vi "AmpCal.vi"(4 "Burst Ct":i8[](array[numeric])=[1, 3, 5, 10, 20], 6 "CA Threshold":i16=62, 8 "File Name In":string, 9 "Voltage Steps":sgl[](array[numeric])=[100.0] format="%_3g", 10 "Motion Settings":T1={"No Motion?"=FALSE, "Motion System"=enum."NI 735x", "Motion Bd ID"=1, "Motion Profile"="SMAC1", "# Axis"=1, "Reverse Z axis?"=TRUE, "SMAC Axis"=0, "scan pair"=enum."y-(x) scan", "RT fps"=6.0, "Steps per mm"=[1000, 1000, 1000, 1000], "Motor Parameters"={"velocity ct/s"=[10000.0, 10000.0, 10000.0, 50000.0], "accel ct/s^2"=[50000.0, 50000.0, 50000.0, 200000.0]}, "One Way Scan"=FALSE, "Reverse One Way Scan"=FALSE, "Global Position (mm)"=[], "Plane"=0, "Distance between\nscan lines (um)"=0.0, "Distance between\nscan planes (um)"=0.0, "number of scan planes"=1, "Total steps in line"=0, "Xtra plane\ndistance  (um)"=100, "Xtra planes "=1, "Add Axis"=FALSE, "overshoot cts"=200, "BKPT Shift"=0, "Scan Start Time (ms)"=0, "ESP VISA"="GPIB::1::INSTR", "3rd Axis"=1, "GL Ref Out"=refnum, "Galil Address"=""} {"3rd Axis" items=["x", "y", "z", "w"]; "Xtra planes" min=1; "Xtra plane\ndistance  (um)" min=0; "Distance between\nscan planes (um)" format="%.2f"; "Distance between\nscan lines (um)" format="%.2f"; "SMAC Axis" items=["None"=0, "Axis 1"=1, "Axis 2"=2, "Axis 3"=3, "Axis 4"=4, "Axis 5"=5, "Axis 6"=6, "Axis 7"=7, "Axis 8"=8, "Vector Space 1"=17, "Vector Space 2"=18, "Vector Space 3"=19, "Vector Space 4"=20]; "Motion Bd ID" min=1 max=32 step=1}, 11 "Digitizer Settings":T5={"Digitizer delay (us) "=0.0, "rf points per line"=2048, "lines per plane"=128, "Samp Rate (Hz)"=100000000.0, "Additional dig delay (us)"=0.0, "Voltage Scale"=0.4, "Pre-Looks"=0, "Offset delay (us)"=0.0, "bits A/D"=8, "Avg Num"=1, "DigTimeOut"=5.0, "Rel Dig Delay"=0.0, "Dig Ch"=0, "LeCroyCluster"={"LeCroy Channels"=[TRUE, FALSE, FALSE, FALSE], "LC read pt offset"=0.0, "Sweep Avg"=FALSE}, "Main Digitizer"=enum."NI Digitizer", "Dig Config"=enum."Single channel", "Digitizer ID Cluster"={"Acqiris/Alazar/SP ID"=[], "NI Instr Handles"=[], "LeCroy VISA"="", "GaGe Handle"={"Handle"=0, "Sample size"=0, "Resolution"=0, "Offset"=0, "Channels"=0, "Boards"=0}, "ATS Ref"="ATS9350", "Acqiris Address"=["PCI::INSTR0"], "ADQRef"=refnum, "adq_cu_ptr"=refnum}, "Trigger Settings"={"Trig Source"=1, "Trig Coupling"=0, "Trig Slope"=0, "Level (mV)"=1500.0}, "Bulk Acq"=FALSE, "Bulk Start Indexes"=[], "Data Ref RF"=refnum, "NI ID/Channel"=[], "Total Dig CH"=5, "Xtra Ann Trig delay (us)"=10.0, "Fix Z Delay?"=FALSE, "One Way Transmission?"=FALSE, "Data Ref Log"=refnum} {"Trigger Settings"."Trig Slope" items=["Positive", "Negative"]; "Trigger Settings"."Level (mV)" format="%.2f"; "Trigger Settings"."Trig Coupling" items=["DC 1 MOhm", "AC 1 MOhm", "DC 50 Ohm", "AC 50 Ohm"]; "Trigger Settings"."Trig Source" items=["Chan 1", "External"]; "Rel Dig Delay" format="%.2f"; "DigTimeOut" format="%.2f"; "Avg Num" min=1; "Offset delay (us)" format="%.2f"; "Additional dig delay (us)" format="%.2f"; "Digitizer delay (us)" format="%.2f"}) -> (1 "Scan Params":T9, 2 "low %":dbl, 3 "clip%":dbl)   [LabVIEW 2022 SP3]
uses:
  ScanningControl/Motion Controllers/-MotionRoutines/MotionGlobals.vi
  <instrlib>/Acqiris Dx/Acqiris Dx.lvlib
  Instance           7 16Saved   Contrast .vi
  Instance           8 16Saved   Contrast .vi
  ScanningControl/Digitizers/Acqiris/-AcqirisRoutines/VScaleInfoAcq.vi
  <instrlib>/niScope/Acquire/Fetch/niScope Multi Fetch Binary 8.vi
  ScanningControl/Digitizers/NI Digitizer/-NI Digitizer VI Library/VScaleInfoNI.vi
  <vilib>/Utility/file.llb/Write To Spreadsheet File (string).vi
  <vilib>/Utility/file.llb/Read From Spreadsheet File (string).vi
  <vilib>/Utility/file.llb/Write To Spreadsheet File (I64).vi
  ScanningControl/Digitizers/-DigitizerRoutines/DigitizerSettings.ctl
  ScanningControl/Digitizers/-DigitizerRoutines/DigitizerID.ctl
  ScanningControl/Digitizers/-DigitizerRoutines/Digitizer.ctl
  ScanningControl/Motion Controllers/NI_controller/-NI_MotionRoutines/MotionSys.ctl
  ScanningControl/Motion Controllers/-MotionRoutines/ScanAxis.ctl
  ScanningControl/Motion Controllers/NI_controller/-NI_MotionRoutines/MotionParameters.ctl
  ScanningControl/Digitizers/-DigitizerRoutines/DigConfig.ctl
  ScanningControl/Motion Controllers/-MotionRoutines/3rdAxis.ctl
  C:/Windows/System32/ADQAPI_dotNet_helper.dll
panel:
  out "try":i32=100
  # "1-D and 2-D B scan settings"
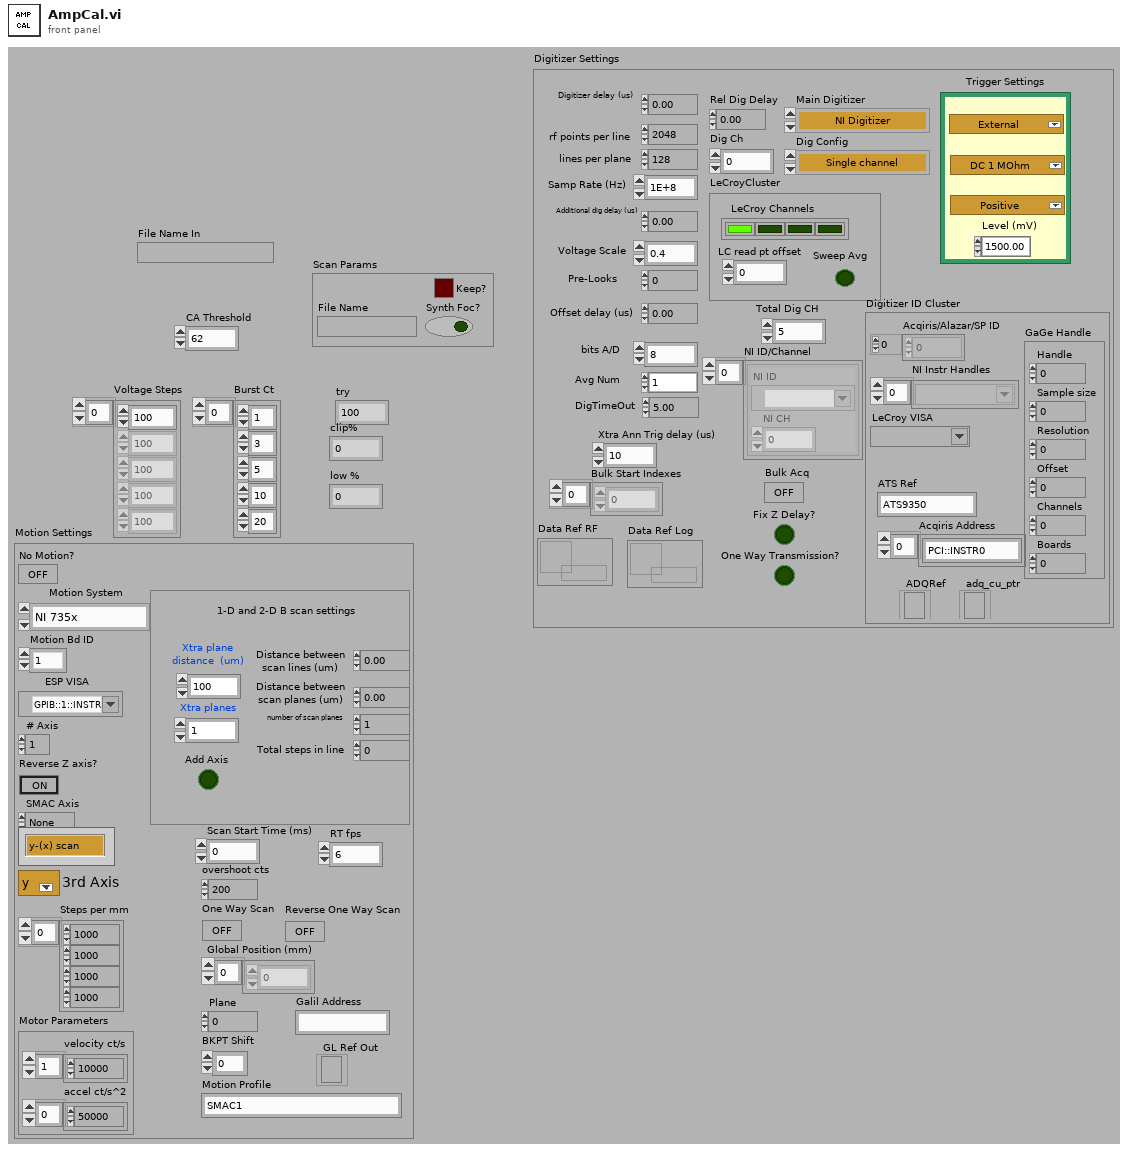
[diagram p1: front panel]
types:
  T1 = typedef "MotionParameters.ctl" = cluster{"No Motion?":bool, "Motion System":T2, "Motion Bd ID":u8, "Motion Profile":string, "# Axis":i8, "Reverse Z axis?":bool, "SMAC Axis":u16, "scan pair":T3, "RT fps":sgl, "Steps per mm":i32[], "Motor Parameters":cluster{"velocity ct/s":dbl[], "accel ct/s^2":dbl[]}, "One Way Scan":bool, "Reverse One Way Scan":bool, "Global Position (mm)":dbl[], "Plane":i32, "Distance between\nscan lines (um)":sgl, "Distance between\nscan planes (um)":sgl, "number of scan planes":i32, "Total steps in line":i32, "Xtra plane\ndistance  (um)":i32, "Xtra planes ":i32, "Add Axis":bool, "overshoot cts":i32, "BKPT Shift":i32, "Scan Start Time (ms)":u32, "ESP VISA":refnum<visa-resource-name>, "3rd Axis":T4, "GL Ref Out":refnum<k7>, "Galil Address":string}
  T2 = typedef "MotionSys.ctl" = enum16{"MM3000", "NI 735x", "Newport ESP", "No Motion Card", "Galil"}
  T3 = typedef "ScanAxis.ctl" = enum16{"y-(x) scan", "x-(y) scan", "z-(x) scan", "z-(y) scan", "y-(z) scan", "x-(z) scan", "w-(x) scan", "w-(y) scan", "w-(z) scan", "x-(w) scan", "y-(w) scan", "z-(w) scan"}
  T4 = typedef "3rdAxis.ctl" = u16
  T5 = typedef "DigitizerSettings.ctl" = cluster{"Digitizer delay (us) ":dbl, "rf points per line":i32, "lines per plane":i32, "Samp Rate (Hz)":dbl, "Additional dig delay (us)":dbl, "Voltage Scale":dbl, "Pre-Looks":i32, "Offset delay (us)":dbl, "bits A/D":i8, "Avg Num":i32, "DigTimeOut":sgl, "Rel Dig Delay":sgl, "Dig Ch":i32, "LeCroyCluster":cluster{"LeCroy Channels":bool[], "LC read pt offset":dbl, "Sweep Avg":bool}, "Main Digitizer":T6, "Dig Config":T7, "Digitizer ID Cluster":T8, "Trigger Settings":cluster{"Trig Source":u16, "Trig Coupling":u16, "Trig Slope":u16, "Level (mV)":dbl}, "Bulk Acq":bool, "Bulk Start Indexes":i32[], "Data Ref RF":refnum<data-value>, "NI ID/Channel":cluster{"NI ID":refnum<k15>, "NI CH":i32}[], "Total Dig CH":i32, "Xtra Ann Trig delay (us)":dbl, "Fix Z Delay?":bool, "One Way Transmission?":bool, "Data Ref Log":refnum<data-value>}
  T6 = typedef "Digitizer.ctl" = enum16{"Acqiris Digitizer", "NI Digitizer", "LeCroy", "GaGe", "AlazarTech", "No Digitizer", "Teledyne"}
  T7 = typedef "DigConfig.ctl" = enum16{"Single channel", "2 Chans w/ 2 Acqiris", "2 Chans w/ 1 Acqiris", "5-CH Pulser New", "5-CH pulser w/ ann array", "5-pass style ann array", "Empty"}
  T8 = typedef "DigitizerID.ctl" = cluster{"Acqiris/Alazar/SP ID":u32[], "NI Instr Handles":refnum<k15>[], "LeCroy VISA":refnum<visa-resource-name>, "GaGe Handle":cluster{"Handle":u32, "Sample size":u32, "Resolution":i32, "Offset":i32, "Channels":u32, "Boards":u32}, "ATS Ref":string, "Acqiris Address":string[], "ADQRef":refnum<k24>, "adq_cu_ptr":refnum<k24>}
  T9 = cluster{"File Name":string, "Keep?":bool, "Synth Foc?":bool}
  T10 = cluster{"Voltage Scale":i16, "Offset":dbl, "Coupling":u16}
  T11 = cluster{"actualSamples":i32, "absoluteInitialX":dbl, "relativeInitialX":dbl, "xIncrement":dbl, "offset":dbl, "gain":dbl, "reserved1":dbl, "reserved2":dbl}[]
  T12 = cluster{"actualSamples":i32, "absoluteInitialX":dbl, "relativeInitialX":dbl, "xIncrement":dbl, "offset":dbl, "gain":dbl, "reserved1":dbl, "reserved2":dbl}
  T13 = cluster{"Voltage Scale":dbl, "Offset":dbl, "Coupling":u16}
  T14 = cluster{sgl, "Gain [dB]  ":sgl, "Atten (dB)":sgl}
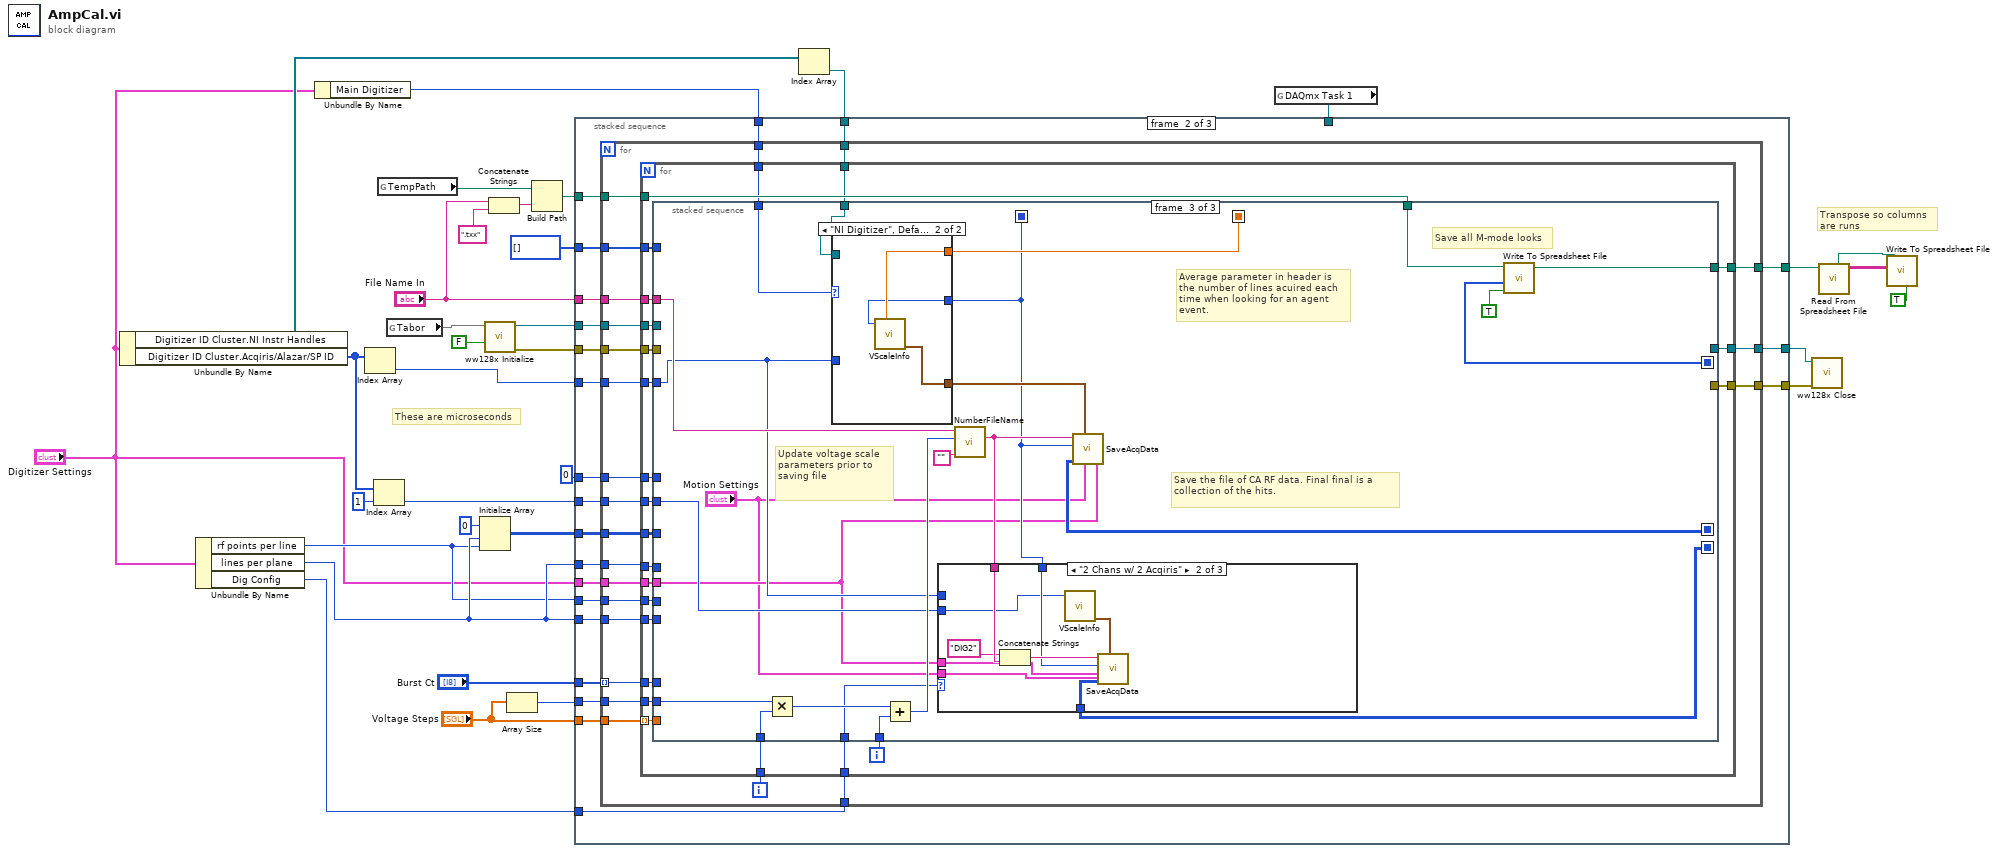
[diagram p0: block diagram]
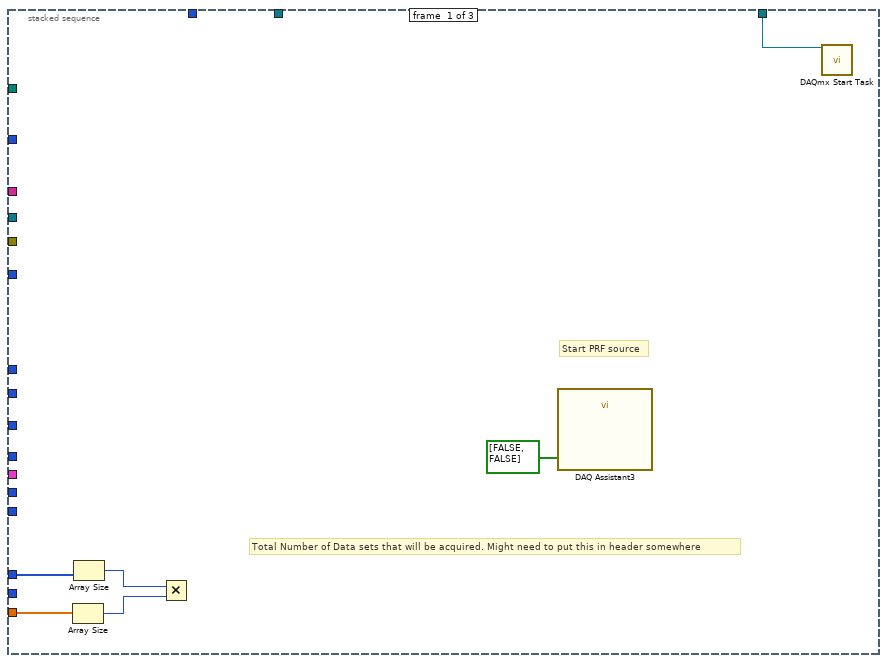
[diagram p2: hidden frame]
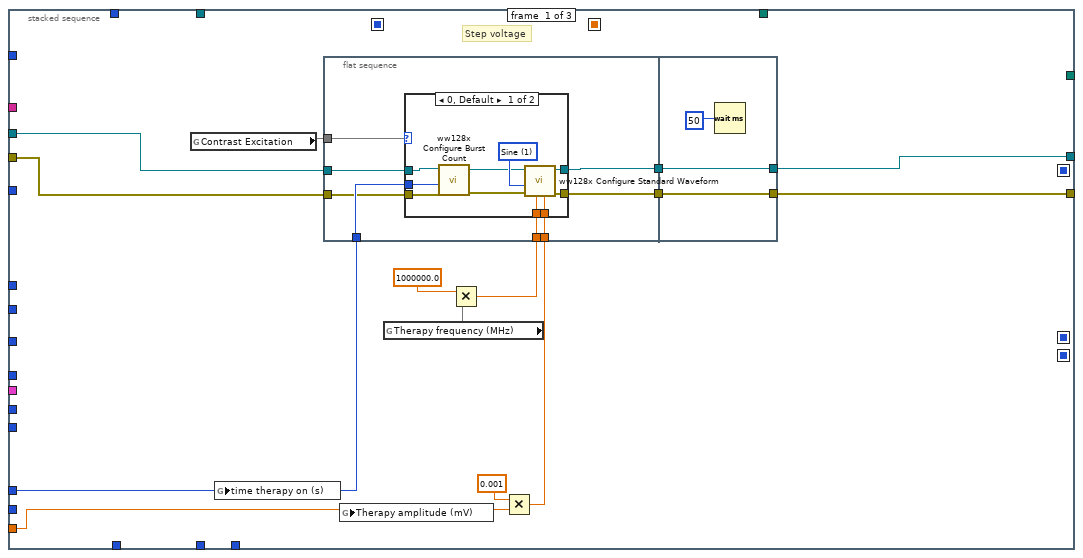
[diagram p3: hidden frame]
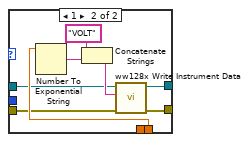
[diagram p4: hidden frame]
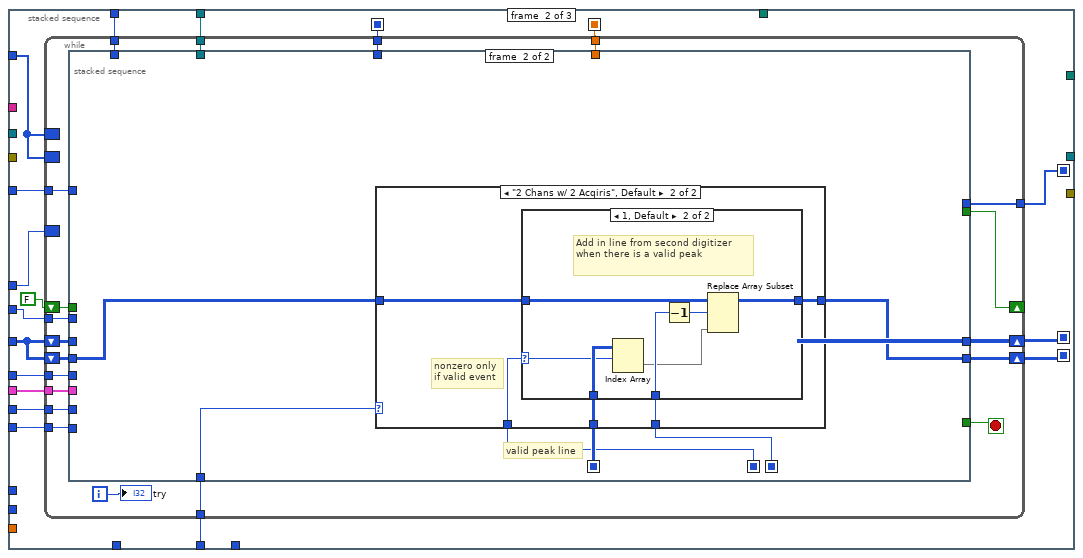
[diagram p5: hidden frame]
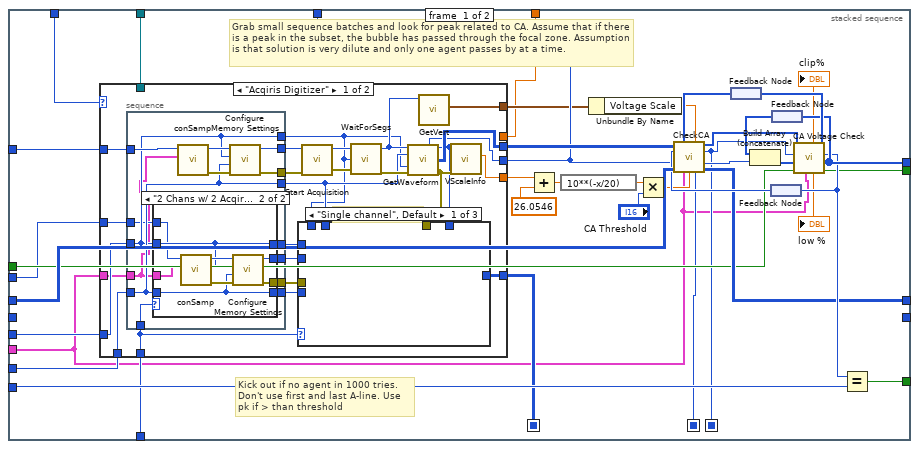
[diagram p6: hidden frame]
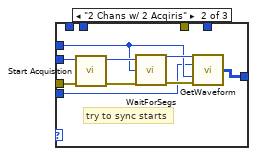
[diagram p7: hidden frame]
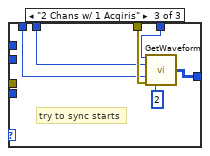
[diagram p8: hidden frame]
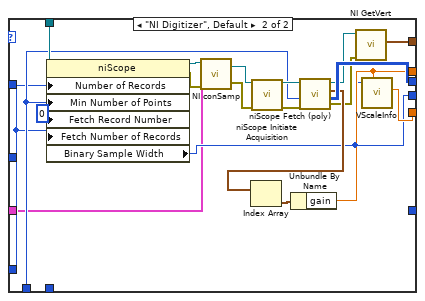
[diagram p10: hidden frame]
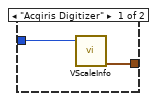
[diagram p13: hidden frame]
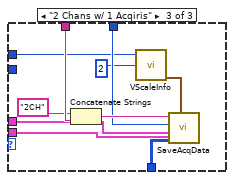
[diagram p15: hidden frame]
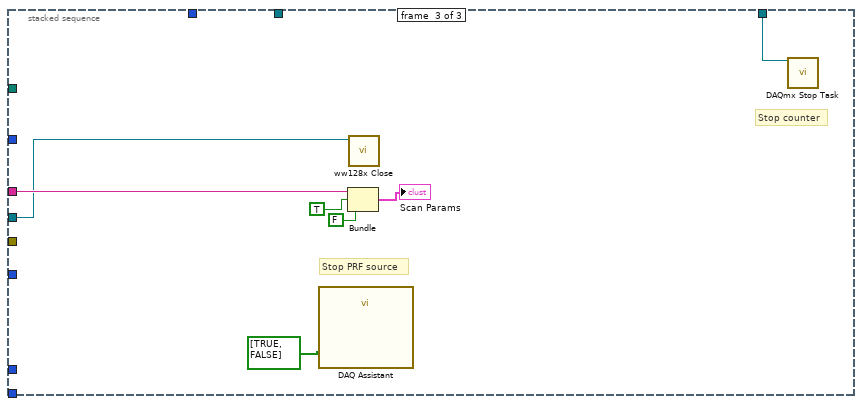
[diagram p16: hidden frame]
diagram:
  # "Transpose so columns are runs"
  # "These are microseconds"
  n1 = Unbundle By Name("Digitizer Settings") -> ("Digitizer ID Cluster.NI Instr Handles"=w9:refnum<k15>[], "Digitizer ID Cluster.Acqiris/Alazar/SP ID"=w8:u32[])
  n2 = Unbundle By Name("Digitizer Settings") -> ("rf points per line"=w4:i32, "lines per plane"=w5:i32, "Dig Config"=w1:T7)
  n3 = Unbundle By Name("Digitizer Settings") -> ("Main Digitizer"=w2:T6)
  n4 = Index Array(array=w8) -> (element=w10:u32)  [unwired: 1 in]
  n5 = Index Array(array=w8, index=1) -> (element=w6:u32)
  n6 = global read "MotionGlobals.vi" "TempPath"() -> (w11:path)
  n7 = global read "MotionGlobals.vi" "Tabor"() -> (w13)
  n8 = Initialize Array(i16 0, w5, w4) -> (w33:i16[][])
  n9 = call <instrlib>:"ww128x Initialize.vi"("reset device (Yes)"=FALSE ("reset device"), "resource name"=w13) -> ("error out"=w15:errorcluster, "instrument handle out"=w14:refnum<k15>)  [unwired: 2 in, 6 out]
  n10 = Concatenate Strings("File Name In", ".txx") -> (w21:string)
  n11 = Array Size(array="Voltage Steps") -> (size(s)=w28:i32)
  n12 = Build Path(base path=w11, name or relative path=w21) -> (appended path=w19:path)
  n13 = Index Array(array=w9) -> (element=w12:refnum<k15>)  [unwired: 1 in]
  n14 = global read "MotionGlobals.vi" "DAQmx Task 1"() -> (w31:refnum<k21>)
  n15 = stacked-sequence {
    tunnel: w10 -> [_ w62 _]
    tunnel: w4 -> [_ w61 _]
    tunnel: w5 -> [_ w60 _]
    tunnel: w33 -> [_ w59 _]
    tunnel: 0 -> [_ w58 _]
    tunnel: w5 -> [_ w57 _]
    tunnel: "File Name In" -> [_ w56 w382]
    tunnel: w31 -> [w40 _ w385]
    tunnel: i32[] [] -> [_ w55 _]
    tunnel: "Burst Ct" -> [w37 w54 _]
    tunnel: "Voltage Steps" -> [w38 w53 _]
    tunnel: w28 -> [_ w52 _]
    tunnel: [_ w51 _] -> w27
    tunnel: w19 -> [_ w50 _]
    tunnel: [_ w49 _] -> w18
    tunnel: [_ w48 _] -> w17
    tunnel: w15 -> [_ w47 _]
    tunnel: w14 -> [_ w46 w380]
    tunnel: w2 -> [_ w45 _]
    tunnel: w12 -> [_ w44 _]
    tunnel: w6 -> [_ w43 _]
    tunnel: "Digitizer Settings" -> [_ w42 _]
    tunnel: w1 -> [_ w41 _]
    frame #0 {
      # "Total Number of Data sets that will be acquired. Might need to put this in header somewhere"
      # "Start PRF source"
      n16 = Array Size(array=w38) -> (size(s)=w35:i32)
      n17 = Array Size(array=w37) -> (size(s)=w36:i32)
      n18 = Multiply(x=w36, y=w35) -> ()  [unwired: 1 out]
      n19 = call "DAQ Assistant3"("data"=bool[] [FALSE, FALSE]) -> ()  [unwired: 3 in, 16 out]
      n20 = call <vilib>:"DAQmx Start Task.vi"("task/channels in"=w40) -> ()  [unwired: 1 in, 14 out]
    }
    frame #1 {
      n21 = for {
        tunnel: w62 -> [w85]
        tunnel: w61 -> [w84]
        tunnel: w60 -> [w83]
        tunnel: w59 -> [w82]
        tunnel: w58 -> [w81]
        tunnel: w57 -> [w80]
        tunnel: w56 -> [w79]
        tunnel: w55 -> [w78]
        tunnel: w54 -> [w77] mode=indexing
        tunnel: w53 -> [w76]
        tunnel: w52 -> [w75]
        tunnel: [w73] -> w51
        tunnel: w50 -> [w72]
        tunnel: [w71] -> w49
        tunnel: [w70] -> w48
        tunnel: w47 -> [w69]
        tunnel: w46 -> [w68]
        tunnel: w45 -> [w67]
        tunnel: w44 -> [w66]
        tunnel: w41 -> [w65]
        tunnel: w43 -> [w64]
        tunnel: w42 -> [w63]
        i -> [w74]
        n22 = for {
          tunnel: w85 -> [w109]
          tunnel: w83 -> [w108]
          tunnel: w84 -> [w107]
          tunnel: w82 -> [w106]
          tunnel: w81 -> [w105]
          tunnel: w80 -> [w104]
          tunnel: w79 -> [w103]
          tunnel: w78 -> [w102]
          tunnel: w77 -> [w101]
          tunnel: w76 -> [w100] mode=indexing
          tunnel: w75 -> [w99]
          tunnel: w74 -> [w98]
          tunnel: [w96] -> w73
          tunnel: w72 -> [w95]
          tunnel: [w94] -> w71
          tunnel: [w93] -> w70
          tunnel: w69 -> [w92]
          tunnel: w68 -> [w91]
          tunnel: w67 -> [w90]
          tunnel: w66 -> [w89]
          tunnel: w65 -> [w88]
          tunnel: w64 -> [w87]
          tunnel: w63 -> [w86]
          i -> [w97]
          n23 = stacked-sequence {
            seq-local: [_ w166 _] -> [_ _ w353]
            seq-local: [_ w164 _] -> [_ _ w335]
            seq-local: [_ w158 _] -> [_ _ w346]
            seq-local: [_ w156 _] -> [_ _ w341]
            seq-local: [_ w155 _] -> [_ _ w336]
            tunnel: w109 -> [_ w169 w337]
            tunnel: w108 -> [_ w168 _]
            tunnel: w107 -> [_ w170 _]
            tunnel: w106 -> [_ w159 _]
            tunnel: w105 -> [_ w167 _]
            tunnel: w104 -> [_ w157 _]
            tunnel: w103 -> [_ _ w354]
            tunnel: w102 -> [_ w165 _]
            tunnel: w101 -> [w117 _ _]
            tunnel: w100 -> [w118 _ _]
            tunnel: w99 -> [_ _ w352]
            tunnel: w98 -> [_ _ w351]
            tunnel: w97 -> [_ _ w350]
            tunnel: w95 -> [_ _ w347]
            tunnel: [_ _ w344] -> w96
            tunnel: [w114 _ _] -> w94
            tunnel: [w112 _ _] -> w93
            tunnel: w92 -> [w111 _ _]
            tunnel: w91 -> [w110 _ _]
            tunnel: w90 -> [_ w162 w339]
            tunnel: w89 -> [_ w161 w340]
            tunnel: w88 -> [_ w160 w343]
            tunnel: w87 -> [_ w154 w334]
            tunnel: w86 -> [_ w153 w333]
            frame #0 {
              # "Step voltage"
              n24 = global read "MotionGlobals.vi" "Contrast Excitation"() -> (w116)
              n25 = global write "MotionGlobals.vi" "time therapy on (s)"(w117) -> ()
              n26 = flat-sequence {
                tunnel: w117 -> [w128]
                tunnel: w120 -> [w131]
                tunnel: w119 -> [w130]
                tunnel: w116 -> [w129]
                tunnel: [w127] -> w115
                tunnel: [w126] -> w113
                tunnel: w111 -> [w125]
                tunnel: w110 -> [w124]
                tunnel: w115 -> [w151]
                tunnel: [w151] -> w114
                tunnel: [w150] -> w112
                tunnel: w113 -> [w150]
                frame #0 {
                  n27 = case shown="0, Default" w129 {
                    tunnel: [w141 w149] -> w126
                    tunnel: w131 -> [w140 w145]
                    tunnel: w130 -> [w139 _]
                    tunnel: w128 -> [w135 _]
                    tunnel: [w134 w144] -> w127
                    tunnel: w125 -> [w132 w143]
                    tunnel: w124 -> [w133 w142]
                    frame 0, Default {
                      w138 = 1 items=["Sine"=1, "Square"=2, "Triangle"=3, "Ramp Up"=4, "Ramp Down"=5, "DC"=6, "Ramp"=1001, "Pulse"=1005, "Sync"=1002, "Gaussian"=1003, "Exponential"=1004, "Noise"=1006] ("waveform")
                      n28 = call <instrlib>:"ww128x Configure Burst Count.vi"("error in (no error)"=w132, "burst count (2)"=w135, "instrument handle"=w133) -> ("error out"=w137:errorcluster, "instrument handle out"=w136:refnum<k15>)  [unwired: 1 in, 6 out]
                      n29 = call <instrlib>:"ww128x Configure Standard Waveform.vi"("amplitude"=w140, "frequency"=w139, "error in (no error)"=w137, "waveform"=w138, "instrument handle"=w136) -> ("error out"=w134:errorcluster, "instrument handle out"=w141:refnum<k15>)  [unwired: 3 in, 2 out]
                    }
                    frame 1 {
                      n30 = Number To Exponential String(number=w145) -> (E-format string=w147:string)  [unwired: 3 out]
                      n31 = Concatenate Strings("VOLT" ("string"), w147) -> (w146:string)
                      n32 = call <instrlib>:"ww128x Write Instrument Data.vi"("error in (no error)"=w143, "write buffer"=w146, "instrument handle"=w142) -> ("error out"=w144:errorcluster, "instrument handle out"=w149:refnum<k15>)  [unwired: 7 out]
                    }
                  }
                }
                frame #1 {
                  n33 = Wait (ms)(milliseconds to wait=50) -> ()  [unwired: 1 out]
                }
              }
              n34 = global write "MotionGlobals.vi" "Therapy amplitude (mV)"(w118) -> ()
              n35 = global read "MotionGlobals.vi" "Therapy frequency (MHz)"() -> (w122)
              n36 = Multiply(x=1000000.0, y=w122) -> (x*y=w119:dbl)
              n37 = Multiply(x=0.001, y=w118) -> (x*y=w120:dbl)
            }
            frame #1 {
              n38 = while {
                tunnel: w170 -> [w187]
                tunnel: w169 -> [w190]
                tunnel: w168 -> [w186]
                shift-right: [w184] -> w166
                shift-left: w159 -> [w189]
                tunnel: w157 -> [w176]
                border: w167 -> [_]
                border: w165 -> [_]
                border: w165 -> [_]
                tunnel: [w180] -> w164
                shift-right: [w182] -> _
                shift-left: FALSE -> [w183]
                tunnel: w162 -> [w181]
                tunnel: w161 -> [w179]
                tunnel: w160 -> [w178]
                shift-right: [w174] -> w156
                shift-left: w159 -> [w175]
                tunnel: [w185] -> w158
                tunnel: [w173] -> w155
                tunnel: w154 -> [w172]
                tunnel: w153 -> [w171]
                i -> [w177]
                stop <- w188 stop-if-true
                n39 = stacked-sequence {
                  seq-local: [w196 _] -> [_ w315]
                  seq-local: [w195 _] -> [_ w317]
                  seq-local: [w194 _] -> [_ w313]
                  tunnel: w190 -> [w229 _]
                  tunnel: w189 -> [w228 _]
                  tunnel: [w227 _] -> w188
                  tunnel: w176 -> [w226 _]
                  tunnel: w187 -> [w225 _]
                  tunnel: w186 -> [w224 _]
                  tunnel: [w217 _] -> w185
                  tunnel: [w215 _] -> w184
                  tunnel: w183 -> [w206 _]
                  tunnel: [w205 _] -> w182
                  tunnel: w181 -> [w203 _]
                  tunnel: [w202 _] -> w180
                  tunnel: w179 -> [w200 _]
                  tunnel: w178 -> [w197 w314]
                  tunnel: w175 -> [_ w316]
                  tunnel: [_ w312] -> w174
                  tunnel: [w193 _] -> w173
                  tunnel: w172 -> [w192 _]
                  tunnel: w171 -> [w191 _]
                  frame #0 {
                    # "Grab small sequence batches and look for peak related to CA. Assume that if there is a peak in the subset, the bubble has passed through the focal zone. Assumption is that solution is very dilute and only one agent passes by at a time."
                    # "Kick out if no agent in 1000 tries. Don't use first and last A-line. Use pk if > than threshold"
                    n40 = case shown="\"Acqiris Digitizer\"" w203 {
                      tunnel: w229 -> [w252 _]
                      tunnel: w225 -> [w244 w299]
                      tunnel: w224 -> [w239 w298]
                      tunnel: [w246 w307] -> w223
                      tunnel: [w232 w293] -> w202
                      tunnel: [w249 w311] -> w201
                      tunnel: [w245 w308] -> w209
                      tunnel: w200 -> [_ w300]
                      tunnel: w197 -> [w238 _]
                      tunnel: [w243 _] -> w196
                      tunnel: [_ w294] -> w193
                      tunnel: w192 -> [w231 _]
                      tunnel: w191 -> [w230 w292]
                      frame "Acqiris Digitizer" {
                        # "2nd digitizer acq"
                        n41 = stacked-sequence {
                          tunnel: w252 -> [w281]
                          tunnel: [w280] -> w251
                          tunnel: [w279] -> w250
                          tunnel: w244 -> [w276]
                          tunnel: [w278] -> w242
                          tunnel: [w277] -> w241
                          tunnel: [w276] -> w234
                          tunnel: [w275] -> w233
                          tunnel: [w273] -> w240
                          tunnel: w239 -> [w275]
                          tunnel: w238 -> [w274]
                          tunnel: [w272] -> w237
                          tunnel: w231 -> [w271]
                          tunnel: w230 -> [w270]
                          frame #0 {
                            n42 = case shown="\"2 Chans w/ 2 Acqiris\"" w274 {
                              tunnel: [_ w291] -> w278
                              tunnel: [_ w288] -> w277
                              tunnel: w276 -> [_ w286]
                              tunnel: w275 -> [_ w287]
                              tunnel: [_ w287] -> w273
                              tunnel: [_ w286] -> w272
                              tunnel: w271 -> [_ w285]
                              tunnel: w270 -> [_ w284]
                              frame "Single channel", Default {
                              }
                              frame "2 Chans w/ 2 Acqiris" {
                                n43 = call "conSamp.vi"("Digitizer Settings"=w284, "InstrumentID"=w285) -> ("error out"=w289:errorcluster, "DUP ID"=w290:u32)  [unwired: 2 in]
                                n44 = call <instrlib>:"Configure Memory Settings.vi"("error in (no error)"=w289, "Number of Samples (1000)"=w286, "Number of Segments (1)"=w287, "Instrument ID"=w290) -> ("error out"=w288:errorcluster, "dup Instrument ID"=w291:u32)  [unwired: 2 out]
                              }
                            }
                            n45 = call "conSamp.vi"("Digitizer Settings"=w270, "InstrumentID"=w281) -> ("error out"=w282:errorcluster, "DUP ID"=w283:u32)  [unwired: 2 in]
                            n46 = call <instrlib>:"Configure Memory Settings.vi"("error in (no error)"=w282, "Number of Samples (1000)"=w276, "Number of Segments (1)"=w275, "Instrument ID"=w283) -> ("error out"=w279:errorcluster, "dup Instrument ID"=w280:u32)  [unwired: 2 out]
                          }
                        }
                        n47 = call <instrlib>:"Start Acquisition.vi"("error in (no error)"=w250, "Instrument ID"=w251) -> ("error out"=w253:errorcluster, "dup Instrument ID"=w254:u32)  [unwired: 2 in]
                        n48 = call "WaitForSegs.vi"("Acqiris ID"=w254, "lines per plane"=w233, "error in"=w253) -> ("dup Instrument ID"=w248:u32, "error out"=w247:errorcluster)  [unwired: 1 in, 2 out]
                        n49 = call "GetWaveform.vi"("Acq ID Out"=w248, "Num Samps"=w234, "Num Segs"=w233, "error in"=w247) -> ("Dig Word Size"=w232:u16, "Acq ID Out"=w235:u32, "Acquired Waveform16 bit"=w246:i16[][], "error out"=w236:errorcluster)  [unwired: 2 in, 6 out]
                        n50 = case shown="\"Single channel\", Default" w238 {
                          tunnel: [_ w263 w269] -> w243
                          tunnel: w242 -> [_ w261 _]
                          tunnel: w241 -> [_ w259 _]
                          tunnel: w240 -> [_ w256 _]
                          tunnel: w237 -> [_ w255 _]
                          tunnel: w236 -> [_ _ w268]
                          tunnel: w235 -> [_ _ w267]
                          tunnel: w234 -> [_ _ w265]
                          tunnel: w233 -> [_ _ w264]
                          frame "Single channel", Default {
                          }
                          frame "2 Chans w/ 2 Acqiris" {
                            # "try to sync starts"
                            n51 = call <instrlib>:"Start Acquisition.vi"("error in (no error)"=w259, "Instrument ID"=w261) -> ("error out"=w258:errorcluster, "dup Instrument ID"=w260:u32)  [unwired: 2 in]
                            n52 = call "WaitForSegs.vi"("Acqiris ID"=w260, "lines per plane"=w256, "error in"=w258) -> ("dup Instrument ID"=w262:u32, "error out"=w257:errorcluster)  [unwired: 1 in, 2 out]
                            n53 = call "GetWaveform.vi"("Acq ID Out"=w262, "Num Samps"=w255, "Num Segs"=w256, "error in"=w257) -> ("Acquired Waveform16 bit"=w263:i16[][])  [unwired: 2 in, 9 out]
                          }
                          frame "2 Chans w/ 1 Acqiris" {
                            # "try to sync starts"
                            n54 = call "GetWaveform.vi"("Acq ID Out"=w267, "Num Samps"=w265, "Num Segs"=w264, "error in"=w268, "Channel"=2) -> ("Acquired Waveform16 bit"=w269:i16[][])  [unwired: 1 in, 9 out]
                          }
                        }
                        n55 = call "GetVert.vi"("InstrumentID"=w248) -> ("V scale"=w249:T10)  [unwired: 3 in, 3 out]
                        n56 = call-poly "VScaleInfo.vi"("Instrument ID"=w235, "error in (no error)"=w236) -> ("vGain (dB)"=w245:dbl)  [unwired: 1 in, 7 out]
                      }
                      frame "NI Digitizer", Default {
                        n57 = property class="niScope"(reference=w300, "Number of Records"=w298, "Min Number of Points"=w299, "Fetch Record Number"=0, "Fetch Number of Records"=w298) -> (reference out=w304:refnum<k15>, error out=w301:errorcluster, "Binary Sample Width"=w293:i32)  [unwired: 1 in]
                        n58 = call "NI conSamp.vi"("error in"=w301, "Digitizer Settings"=w292, "InstrumentID"=w304) -> ("error out"=w302:errorcluster, "DUP ID"=w303:refnum<k15>)  [unwired: 1 in]
                        n59 = call <instrlib>:"niScope Initiate Acquisition.vi"("instrument handle"=w303, "error in"=w302) -> ("instrument handle out"=w310:refnum<k15>, "error out"=w309:errorcluster)  [unwired: 1 in, 11 out]
                        n60 = call-poly <instrlib>:"niScope Fetch (poly).vi"("error in"=w309, "numSamples"=w299, "instrument handle"=w310) -> ("error out"=w295:errorcluster, "wfm"=w307:i8[][], "wfm info"=w297:T11, "instrument handle out"=w305:refnum<k15>)  [unwired: 2 in, 3 out]
                        n61 = Index Array(array=w297) -> (element=w296:T12)  [unwired: 1 in]
                        n62 = Unbundle By Name(w296) -> ("gain"=w294:dbl)
                        n63 = call "NI GetVert.vi"("error in"=w295, "InstrumentID"=w305) -> ("V scale"=w311:T13)  [unwired: 1 in, 4 out]
                        n64 = call-poly "VScaleInfo.vi"("A/D bits"=w293, "gain"=w294) -> ("vGain (dB)"=w308:dbl)  [unwired: 1 in, 7 out]
                      }
                    }
                    n65 = Add(x=w209, y=26.0546) -> (x+y=w208:dbl)
                    n66 = expression code="10**(-x/20)"(w208) -> (w199:dbl)
                    n67 = Unbundle By Name(w201) -> ("Voltage Scale"=w210:dbl)
                    n68 = Multiply(x=w199, y="CA Threshold") -> (x*y=w207:dbl)
                    n69 = feedback #1() -> (w212:i32[])
                    n70 = feedback #2() -> (w222:i32)
                    n71 = call "CheckCA.vi"("data"=w223, "valid peak in"=w212, "Voltage Scale"=w210, "count in"=w222, "Dig Word Size"=w202, "fill array"=w228, "Digitizer Settings"=w191, "CA Threshold"=w207) -> ("valid peak out"=w211:i32[], "count out"=w195:i32, "All peaks"=w221:i32, "valild peak line"=w194:i32, "fill out"=w215:i16[][])  [unwired: 3 in]
                    n72 = feedback #3() -> (w220:i32[])
                    n73 = Build Array (concatenate)(w220, w221) -> (w218:i32[])
                    n74 = call "CA Voltage Check.vi"("Digitizer Settings"=w191, "Up Once?"=w206, "All Peak in"=w218, "count in"=w195, "valid peak in"=w211) -> ("Up Once Out"=w205:bool, "All Peak Out"=w217:i32[], "count out"=w216:i32, "valid peak out"=w219:i32[], "low %"=→"low %":dbl, "clip%"=→"clip%":dbl)  [unwired: 1 in]
                    n75 = feedback-in #1(w219) -> ()
                    n76 = feedback-in #2(w216) -> ()
                    n77 = feedback-in #3(w217) -> ()
                    n78 = Equal?(x=w216, y=w226) -> (x = y?=w227:bool)
                  }
                  frame #1 {
                    # "valid peak line"
                    n79 = case shown="\"2 Chans w/ 2 Acqiris\", Default" w314 {
                      tunnel: w317 -> [_ w323]
                      tunnel: w316 -> [w318 w322]
                      tunnel: w315 -> [_ w321]
                      tunnel: w313 -> [_ w320]
                      tunnel: [w318 w319] -> w312
                      frame "Single channel" {
                      }
                      frame "2 Chans w/ 2 Acqiris", Default {
                        # "nonzero only if valid event"
                        n80 = case shown="1, Default" w320 {
                          selector: w320 -> [_ w326]
                          tunnel: w323 -> [_ w331]
                          tunnel: w322 -> [w324 w330]
                          tunnel: w321 -> [_ w328]
                          tunnel: [w324 w325] -> w319
                          frame 0 {
                          }
                          frame 1, Default {
                            # "Add in line from second digitizer when there is a valid peak"
                            n81 = Index Array(array=w328, index (row)=w326) -> (element=w327:i16[])  [unwired: 1 in]
                            n82 = Decrement(x=w331) -> (x-1=w329:i32)
                            n83 = Replace Array Subset(array=w330, new element=w327, index (row)=w329) -> (w325:i16[][])  [unwired: 1 in]
                          }
                        }
                      }
                    }
                  }
                }
                "try" <- w177
              }
            }
            frame #2 {
              # "Update voltage scale parameters prior to saving file"
              # "Average parameter in header is the number of lines acuired each time when looking for an agent event."
              # "Save all M-mode looks"
              # "Save the file of CA RF data. Final final is a collection of the hits."
              n84 = Multiply(x=w352, y=w351) -> (x*y=w349:i32)
              n85 = case shown="\"NI Digitizer\", Default" w339 {
                tunnel: w340 -> [_ _]
                tunnel: [w357 w360] -> w338
                tunnel: w337 -> [w356 _]
                tunnel: w336 -> [_ w359]
                tunnel: w335 -> [_ w358]
                frame "Acqiris Digitizer" {
                  n86 = call-poly "VScaleInfo.vi"("Instrument ID"=w356) -> ("Voltage Scale"=w357:T14)  [unwired: 2 in, 7 out]
                }
                frame "NI Digitizer", Default {
                  n87 = call-poly "VScaleInfo.vi"("A/D bits"=w358, "gain"=w359) -> ("Voltage Scale"=w360:T14)  [unwired: 8 out]
                }
              }
              n88 = Add(x=w349, y=w350) -> (x+y=w348:i32)
              n89 = call "NumberFileName.vi"("String"="", "File number"=w348, "file name"=w354) -> ("Numbered File"=w342:string)  [unwired: 1 in]
              n90 = case shown="\"2 Chans w/ 2 Acqiris\"" w343 {
                tunnel: w342 -> [_ w369 w379]
                tunnel: w341 -> [_ w366 w376]
                tunnel: w335 -> [_ w365 w375]
                tunnel: w337 -> [_ _ w372]
                tunnel: w334 -> [_ w363 _]
                tunnel: w333 -> [_ w362 w371]
                tunnel: "Motion Settings" -> [_ w361 w370]
                frame "Single channel", Default {
                }
                frame "2 Chans w/ 2 Acqiris" {
                  n91 = Concatenate Strings("DIG2", w369) -> (w367:string)
                  n92 = call-poly "VScaleInfo.vi"("Instrument ID"=w363) -> ("Voltage Scale"=w364:T14)  [unwired: 2 in, 7 out]
                  n93 = call "SaveAcqData.vi"("Digitizer Settings"=w362, "Motion Settings"=w361, "Votage scaling"=w364, "Array"=w366, "Dig Word Size"=w365, "File Name"=w367) -> ()  [unwired: 4 in]
                }
                frame "2 Chans w/ 1 Acqiris" {
                  n94 = Concatenate Strings("2CH", w379) -> (w377:string)
                  n95 = call-poly "VScaleInfo.vi"("Instrument ID"=w372, "Channel (1)"=2) -> ("Voltage Scale"=w374:T14)  [unwired: 1 in, 7 out]
                  n96 = call "SaveAcqData.vi"("Digitizer Settings"=w371, "Motion Settings"=w370, "Votage scaling"=w374, "Array"=w376, "Dig Word Size"=w375, "File Name"=w377) -> ()  [unwired: 4 in]
                }
              }
              n97 = call "SaveAcqData.vi"("Digitizer Settings"=w333, "Motion Settings"="Motion Settings", "Votage scaling"=w338, "Array"=w353, "Dig Word Size"=w335, "File Name"=w342) -> ()  [unwired: 4 in]
              n98 = call-poly <vilib>:"Write To Spreadsheet File.vi"("append to file? (new file:F)"=TRUE ("transpose? (no:F)"), "1D data"=w346, "file path (dialog if empty)"=w347) -> ("new file path (Not A Path if cancelled)"=w344:path)  [unwired: 3 in, 2 out]
            }
          }
        }
      }
    }
    frame #2 {
      # "Stop counter"
      # "Stop PRF source"
      n99 = call "DAQ Assistant"("data"=bool[] [TRUE, FALSE]) -> ()  [unwired: 3 in, 16 out]
      n100 = Bundle("File Name In"=w382, TRUE, FALSE) -> (→"Scan Params":cluster{"File Name In":string, bool, bool})  [unwired: 1 out]
      n101 = call <instrlib>:"ww128x Close.vi"("instrument handle"=w380) -> ()  [unwired: 10 in, 1 out]
      n102 = call <vilib>:"DAQmx Stop Task.vi"("task/channels in"=w385) -> ()  [unwired: 1 in, 14 out]
    }
  }
  n103 = call <instrlib>:"ww128x Close.vi"("error in (no error)"=w18, "instrument handle"=w17) -> ()  [unwired: 10 out]
  n104 = call-poly <vilib>:"Read From Spreadsheet File.vi"("file path (dialog if empty)"=w27) -> ("all rows"=w24:string[][], "new file path (Not A Path if cancelled)"=w25:path)  [unwired: 3 in, 6 out]
  n105 = call-poly <vilib>:"Write To Spreadsheet File.vi"("transpose? (no:F)"=TRUE, "2D data"=w24, "file path (dialog if empty)"=w25) -> ()  [unwired: 3 in, 3 out]
